vi "Read Source.vi"(8 "error in (no error)":errorcluster, 11 "Transition in":refnum<class "Transition.lvclass">) -> (0 "error out":errorcluster, 2 "State Machine.lvlib:State.lvlib:State.lvclass":refnum<class "State.lvclass">, 3 "Transition out":refnum<class "Transition.lvclass">)   [LabVIEW 2024, in "Transition.lvlib" / "Transition.lvclass"]
uses:
  Transition.lvclass
  State/State/State.lvclass
  Transition.lvclass/Transition.ctl
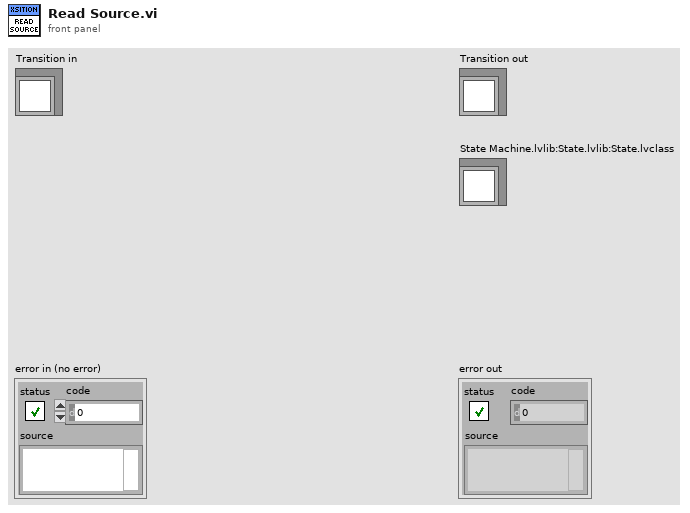
[diagram p1: front panel]
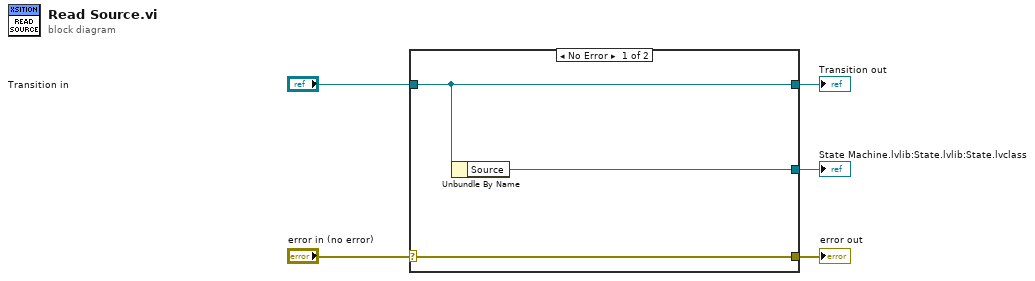
[diagram p0: block diagram]
diagram:
  n1 = case shown="No Error" "error in (no error)" {
    selector: "error in (no error)" -> [w8 w9]
    tunnel: [w8 w9] -> w4
    tunnel: [w7 w10] -> w2
    tunnel: "Transition in" -> [w7 w10]
    tunnel: [w6 _] -> w1
    frame No Error {
      n2 = Unbundle By Name(w7) -> ("Source"=w6:refnum<class "State.lvclass">)
    }
    frame Error {
    }
  }
  "error out" <- w4
  "Transition out" <- w2
  "State Machine.lvlib:State.lvlib:State.lvclass" <- w1
